vi "Write configuration.vi"(8 "error in":errorcluster, 10 "configuration":refnum<class "NISE_CEF_serializable configuration.lvclass">, 11 "Add Module editor node in":refnum<class "Add Module editor node.lvclass">) -> (0 "error out":errorcluster, 3 "Add Module editor node out":refnum<class "Add Module editor node.lvclass">)   [LabVIEW 2018, in "Add Module editor node.lvclass"]
uses:
  Add Module editor node.lvclass
  <vilib>/NI/Configuration Framework/serializable configuration/NISE_CEF_serializable configuration.lvclass
  module/configuration/Add Module configuration.lvclass
  Add Module editor node.lvclass/Add Module editor node.ctl
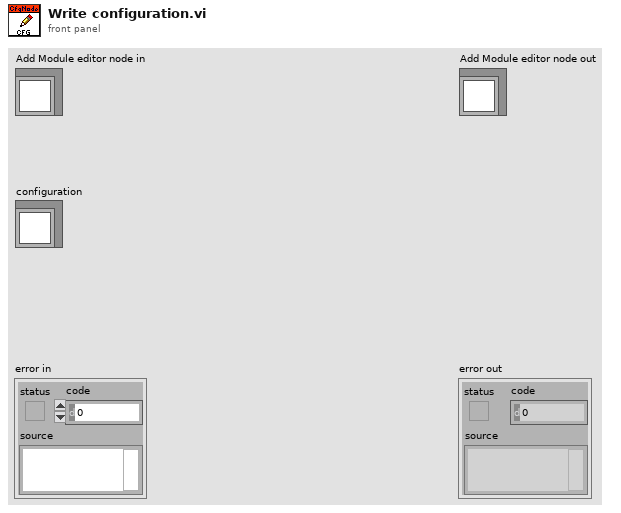
[diagram p1: front panel]
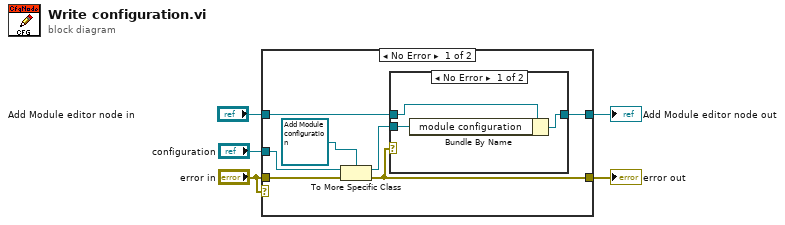
[diagram p0: block diagram]
diagram:
  n1 = case shown="No Error" "error in" {
    tunnel: "error in" -> [w12 w18]
    tunnel: "Add Module editor node in" -> [w11 w17]
    tunnel: [w10 w17] -> w4
    tunnel: [w6 w18] -> w3
    tunnel: "configuration" -> [w9 _]
    frame No Error {
      n2 = To More Specific Class(target class=refnum<class "Add Module configuration.lvclass"> refnum ("module configuration"), reference=w9, error in=w12) -> (specific class reference=w7:refnum<class "Add Module configuration.lvclass">, error out=w6:errorcluster)
      n3 = case shown="No Error" w6 {
        tunnel: w11 -> [w15 w16]
        tunnel: [w14 w16] -> w10
        tunnel: w7 -> [w13 _]
        frame No Error {
          n4 = Bundle By Name(cluster=w15, "module configuration"=w13) -> (w14:refnum<class "Add Module editor node.lvclass">)
        }
        frame Error {
        }
      }
    }
    frame Error {
    }
  }
  "error out" <- w3
  "Add Module editor node out" <- w4
